vi "Init.vi"(8 "error in (no error)":errorcluster caption="entrée d'erreur (pas d'erreur)", 11 "Class LED Analyser in":refnum<class "Class LED Analyser FEASA.lvclass">) -> (0 "error out":errorcluster caption="sortie d'erreur", 3 "Class LED Analyser Out":refnum<class "Class LED Analyser FEASA.lvclass">)   [LabVIEW 2020, in "Library Instrument & Equipement.lvlib" / "Library LED Analyser.lvlib" / "Class LED Analyser FEASA.lvclass"]
uses:
  Class LED Analyser FEASA.lvclass
  C:/Users/ngarcin/OneDrive - Altyor/Standard TB/Class/LED Analyser/Class Led Analyser (Default)/Class LED Analyser (Default).lvclass
  Class LED Analyser FEASA.lvclass/Class LED Analyser FEASA.ctl
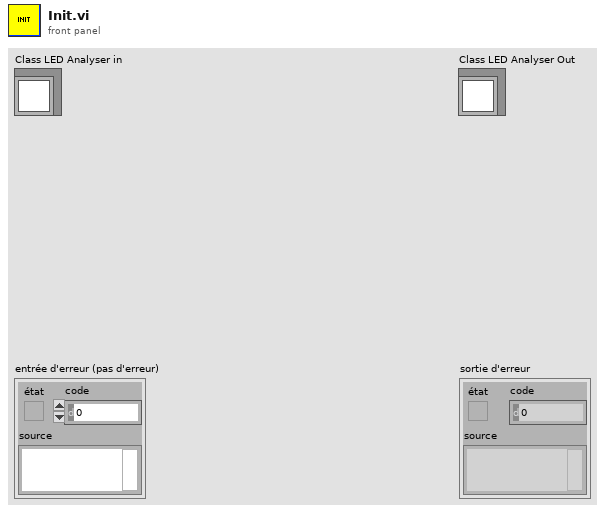
[diagram p1: front panel]
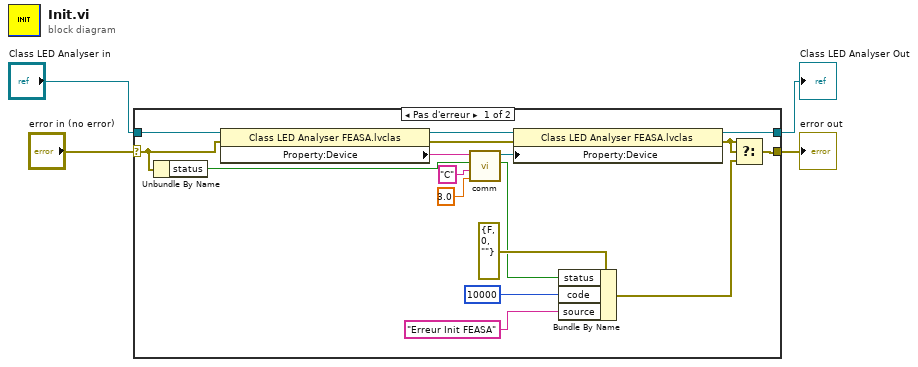
[diagram p0: block diagram]
diagram:
  n1 = case shown="Pas d'erreur" "error in (no error)" {
    selector: "error in (no error)" -> [w8 w23]
    tunnel: [w12 w23] -> w3
    tunnel: [w7 w22] -> w1
    tunnel: "Class LED Analyser in" -> [w11 w22]
    frame No Error {
      n2 = Unbundle By Name(w8) -> ("status"=w18:bool)
      n3 = property class="Class LED Analyser FEASA.lvclas"(reference=w11, error in=w8) -> (reference out=w10:refnum<class "Class LED Analyser FEASA.lvclass">, error out=w9:errorcluster, "Property:Device"=w19:string)
      n4 = call "comm.vi"("Timeout (s)"=3.0, "Command"="C", "Error"=w18, "VISA resource name"=w19) -> ("Error"=w13:bool, "dup VISA resource name"=w5:refnum<visa-resource-name>)  [unwired: 2 in, 2 out]
      n5 = property class="Class LED Analyser FEASA.lvclas"(reference=w10, error in=w9, "Property:Device"=w5) -> (reference out=w7:refnum<class "Class LED Analyser FEASA.lvclass">, error out=w6:errorcluster)
      n6 = Bundle By Name(cluster=errorcluster {"status"=FALSE, "code"=0, "source"=""} ("error IO"), "status"=w13, "code"=10000, "source"="Erreur Init FEASA") -> (w14:errorcluster)
      n7 = Select(t=w6, s=w6, f=w14) -> (s? t:f=w12:errorcluster)
    }
    frame Error {
    }
  }
  "error out" <- w3
  "Class LED Analyser Out" <- w1
